vi "Build Data Blocks.vi"(0 "resampled data":T1, 1 "data block settings":T2={"mode"=enum."IEC 61000-4-30", "cycles per block"=10}, 2 "reset? (F)":bool, 9 "system info in":refnum<class "EP System Info.lvclass">, 11 "error in (no error)":errorcluster) -> (4 "data blocks":T1[](array[typedef]), 10 "system info out":refnum<class "EP System Info.lvclass">, 15 "error out":errorcluster)   [LabVIEW 2014, in "NI_EP_Power Quality.lvlib"]
doc: "Builds even-angle-spaced signals into data blocks. You must use the Resampling for Power Quality VI to resample even-time-spaced voltage and current signals into even-angle-spaced signals. By default, this VI builds data blocks according to IEC 61000-4-30:2008. You can use a customized setting when your application does not follow IEC 61000-4-30:2008.\n\nThis VI supports measuring single-line and multiple-line systems."
uses:
  <vilib>/addons/Electrical Power/PQ/NI_EP_Power Quality.lvlib
  <vilib>/addons/Electrical Power/PQ/Common/Classes/System Info/EP System Info.lvclass
  <vilib>/addons/Electrical Power/PQ/Resampling/Desktop/subVIs/ep_Resampled Data.ctl
  <vilib>/addons/Electrical Power/PQ/Resampling/NI_EP_Resample_Host.lvlib
  <vilib>/addons/Electrical Power/Power Measurement/NI_EP_Power Measurement.lvlib
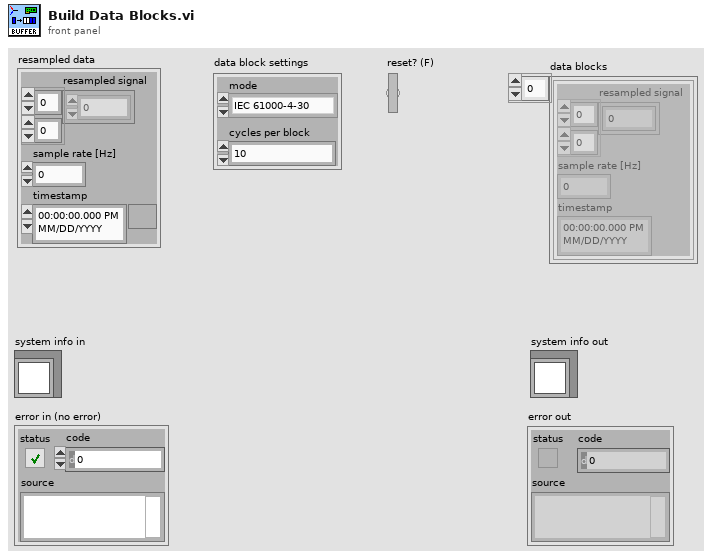
[diagram p1: front panel]
types:
  T1 = typedef "NI_EP_Resample_Host.lvlib/ep_Resampled Data.ctl" = cluster{"resampled signal":dbl[][], "sample rate [Hz]":dbl, "timestamp":timestamp}
  T2 = cluster{"mode":enum16{"IEC 61000-4-30", "Custom"}, "cycles per block":u16}
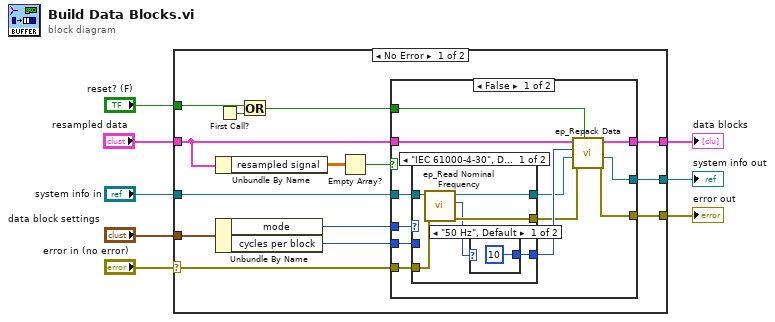
[diagram p0: block diagram]
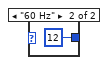
[diagram p2: hidden frame]
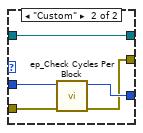
[diagram p3: hidden frame]
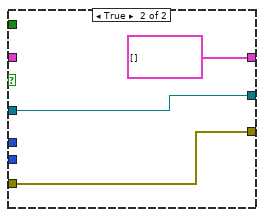
[diagram p4: hidden frame]
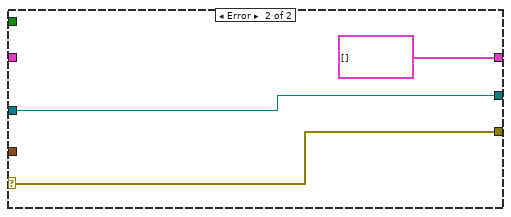
[diagram p5: hidden frame]
diagram:
  n1 = case shown="No Error" "error in (no error)" {
    selector: "error in (no error)" -> [w20 w53]
    tunnel: [w22 T1[] [] ("output data blocks")] -> w7
    tunnel: [w21 w53] -> w6
    tunnel: "system info in" -> [w19 w52]
    tunnel: [w18 w52] -> w4
    tunnel: "data block settings" -> [w17 _]
    tunnel: "reset? (F)" -> [w14 _]
    tunnel: "resampled data" -> [w10 _]
    frame No Error {
      n2 = First Call?() -> (First Call?: T/F=w12:bool)
      n3 = Unbundle By Name(w10) -> ("resampled signal"=w9:dbl[][])
      n4 = Unbundle By Name(w17) -> ("mode"=w16:enum16{"IEC 61000-4-30", "Custom"}, "cycles per block"=w15:u16)
      n5 = Or(x=w14, y=w12) -> (x .or. y?=w13:bool)
      n6 = Empty Array?(array=w9) -> (empty?=w11:bool)
      n7 = case shown="False" w11 {
        tunnel: [w33 T1[] [] ("output data blocks")] -> w22
        tunnel: [w30 w50] -> w21
        tunnel: w20 -> [w24 w50]
        tunnel: w10 -> [w29 _]
        tunnel: w13 -> [w32 _]
        tunnel: w19 -> [w34 w49]
        tunnel: [w31 w49] -> w18
        tunnel: w16 -> [w26 _]
        tunnel: w15 -> [w25 _]
        frame False {
          n8 = case shown="\"IEC 61000-4-30\", Default" w26 {
            tunnel: w34 -> [w40 w47]
            tunnel: [w35 w44] -> w28
            tunnel: [w39 w47] -> w27
            tunnel: w25 -> [_ w45]
            tunnel: w24 -> [w38 w46]
            tunnel: [w37 w43] -> w23
            frame "IEC 61000-4-30", Default {
              n9 = call <vilib>:"ep_Read Nominal Frequency.vi"("error in (no error)"=w38, "system info in"=w40) -> ("error out"=w37:errorcluster, "nominal frequency"=w36:enum16{"50 Hz", "60 Hz"}, "system info out"=w39:refnum<class "EP System Info.lvclass">)  [unwired: 6 in, 1 out]
              n10 = case shown="\"50 Hz\", Default" w36 {
                tunnel: [u16 10 u16 12] -> w35
                frame "50 Hz", Default {
                }
                frame "60 Hz" {
                }
              }
            }
            frame "Custom" {
              n11 = call <vilib>:"ep_Check Cycles Per Block.vi"("error in (no error)"=w46, "cycles per block"=w45) -> ("error out"=w43:errorcluster, "dup cycles per block"=w44:u16)  [unwired: 8 in]
            }
          }
          n12 = call <vilib>:"ep_Repack Data.vi"("reset? (F)"=w32, "error in (no error)"=w23, "system info in"=w27, "cycles per block"=w28, "resampled data"=w29) -> ("error out"=w30:errorcluster, "system info out"=w31:refnum<class "EP System Info.lvclass">, "output data blocks"=w33:T1[])  [unwired: 4 in]
        }
        frame True {
        }
      }
    }
    frame Error {
    }
  }
  "system info out" <- w4
  "error out" <- w6
  "data blocks" <- w7
